vi "old APU + 4 CAMs.vi"() -> ()   [LabVIEW 2013]
uses:
  <vilib>/Platform/TimedLoop/XDataNode/timing_clust.ctl
  <vilib>/Platform/TimedLoop/XDataNode/nitl_modes.ctl
  <vilib>/Platform/TimedLoop/XDataNode/wakeup.ctl
  <userlib>/AES/FPGA/FPGA TypeDefs/aes_FullyCustomTeeth ActionEngine Enum.ctl
  <vilib>/rvi/Emulation/niFpgaSctlEmulationGetInTimedLoop.vi
  <vilib>/rvi/Emulation/niFpgaEmulationReportErrorSimple.vi
  <vilib>/rvi/DataTransferAndStorage/Container/Common/niFpgaContainerGetUniqueNameForEmu.vi
  <vilib>/rvi/DataTransferAndStorage/Container/Common/niFpgaContainerSetEmuInfo.vi
  <vilib>/rvi/eio/common/nirviEmuReportErrorAndStop.vi
  <vilib>/rvi/Emulation/niFpgaGetClockAttributes.vi
  <vilib>/rvi/Emulation/niFpgaCriticalErrorInLSC.vi
  <userlib>/_NI VeriStand FPGA Support/NI VeriStand RIO Library/Custom Device Components/Engine Simulation/Engine Simulation Globals.vi
  <vilib>/rvi/FIFO/Fifo_Resource/nirvififoEmulationReadFpgaImpl.vi
  <vilib>/rvi/eio/common/nirviEmuTemplateMethod_errors.vi
  <vilib>/rvi/Emulation/niFpgaProcessEmulError.vi
  <vilib>/rvi/FIFO/Fifo_Resource/nirvififoEmulationWriteFpgaImpl.vi
  <vilib>/Platform/TimedLoop/XDataNode/XDataNode.xnode
  <vilib>/rvi/LocalResourceManager/LocalResourceManager.xnode
  <vilib>/rvi/DataTransferAndStorage/Container/XNode/niFpgaContainer.xnode
  <vilib>/rvi/FIFO/Fifo_Resource/nirvififoEmulationRead.vi
  <vilib>/eio/EIONode/EIONode.xnode
  <vilib>/rvi/FIFO/Fifo_Resource/nirvififoEmulationWrite.vi
  <vilib>/Platform/TimedLoop/XDataNode/XDNodeRunTimeDep.lvlib
  <userlib>/AES/FPGA/AES FPGA.lvlib
panel:
  in  "FullyCustomTeeth.Cams.Cam1.First Rising?":bool
  in  "FullyCustomTeeth.Cams.Num Angles":u8=2
  in  "FullyCustomTeeth.Cams.Cam1.Offset":u64
  in  "FullyCustomTeeth.Cams.Cam2.Offset":u64
  in  "FullyCustomTeeth.Cams.Cam3.Offset":u64
  in  "FullyCustomTeeth.Cams.Cam4.Offset":u64
  in  "FullyCustomTeeth.Cams.Num Profiles":u8=1
  in  "FullyCustomTeeth.Cams.Cam2.First Rising?":bool
  in  "FullyCustomTeeth.Cams.Cam3.First Rising?":bool
  in  "FullyCustomTeeth.Cams.Cam4.First Rising?":bool
  in  "FullyCustomTeeth.Cams.Cam1.CycleAngle":bool=TRUE
  in  "FullyCustomTeeth.Cams.Cam2.CycleAngle":bool=TRUE
  in  "FullyCustomTeeth.Cams.Cam3.CycleAngle":bool=TRUE
  in  "FullyCustomTeeth.Cams.Cam4.CycleAngle":bool=TRUE
  in  "FullyCustomTeeth.Cams.Data":u64
  in  "FullyCustomTeeth.Cams.Toggle":bool
  in  "APU.Degrees per Tick":u64
  out "APU.Crank Angle":u64
  out "APU.Cycle Angle":u64
  in  "APU.Reset":bool
  in  "APU.Increment Rate":u64
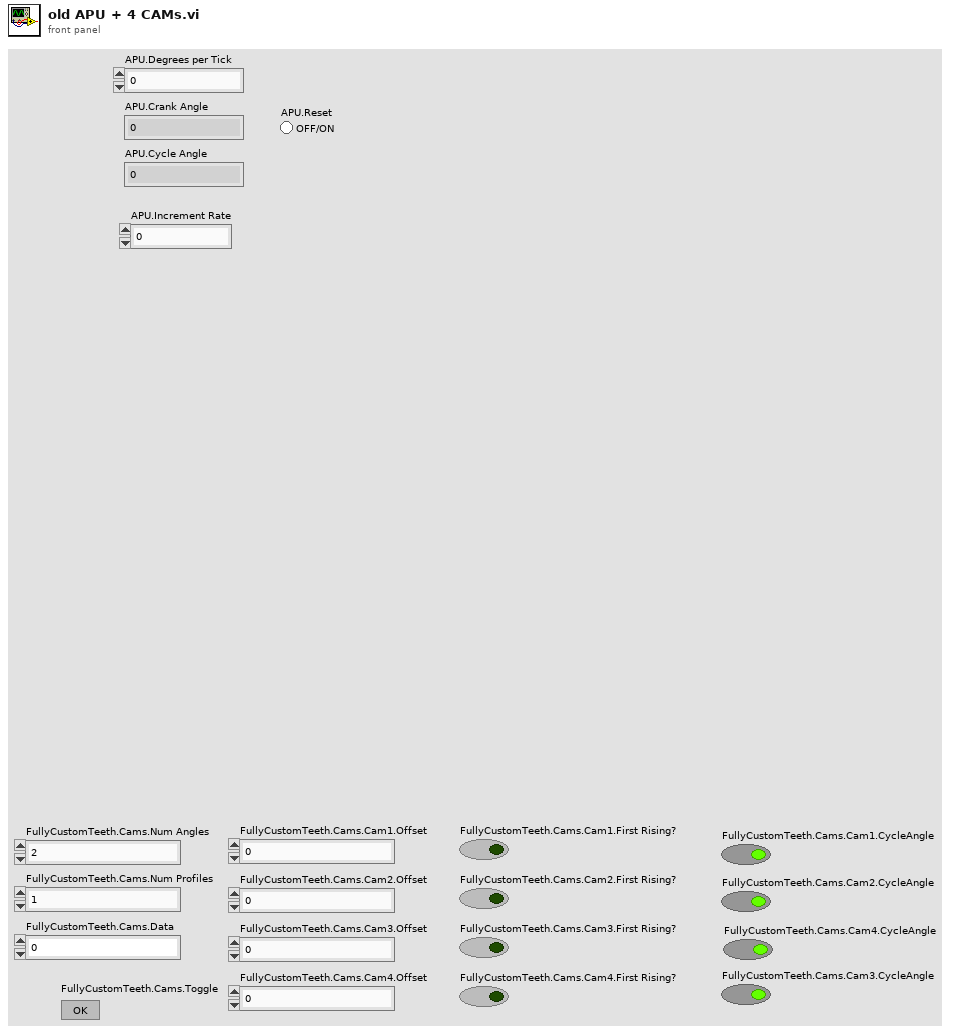
[diagram p1: front panel]
types:
  T1 = typedef "XDNodeRunTimeDep.lvlib/timing_clust.ctl" = cluster{"Expected End [f-1]":u64, "Actual End [f-1]":u64, "Finished Late? [f-1]":bool, "Expected End [i-1]":u64, "Actual End [i-1]":u64, "Finished Late? [i-1]":bool, "Expected Start [i]":u64, "Actual Start [i]":u64, "Expected Start [f]":u64, "Actual Start [f]":u64, "Source Name":string, "Structure Name":string, "Period":i64, "Deadline":i64, "Offset":i64, "Start":i64, "Priority":i32, "Timeout":i32, "Mode":T2, "Wakeup Reason":T3, "Error":errorcluster, "Source Type":string, "Secondary Source Type":string, "Global End Time":u64, "Global Start Time":u64, "Frame Duration":u64, "Iteration Duration":u64, "Assigned CPU":i32, "I/O Scan Engine Mode":u32}
  T2 = typedef "XDNodeRunTimeDep.lvlib/nitl_modes.ctl" = enum32{"No Change", "Process missed periods, maintain original phase", "Discard missed periods, maintain original phase", "Process missed periods, ignore original phase", "Discard missed periods, ignore original phase"}
  T3 = typedef "XDNodeRunTimeDep.lvlib/wakeup.ctl" = enum32{"Normal", "Aborted", "Asynchronous wakeup", "Timing source error", "Timed loop error", "Timeout"}
  T4 = typedef "AES.lvlib/AES FPGA.lvlib/aes_FullyCustomTeeth ActionEngine Enum.ctl" = enum16{"Write Angle", "Update Output"}
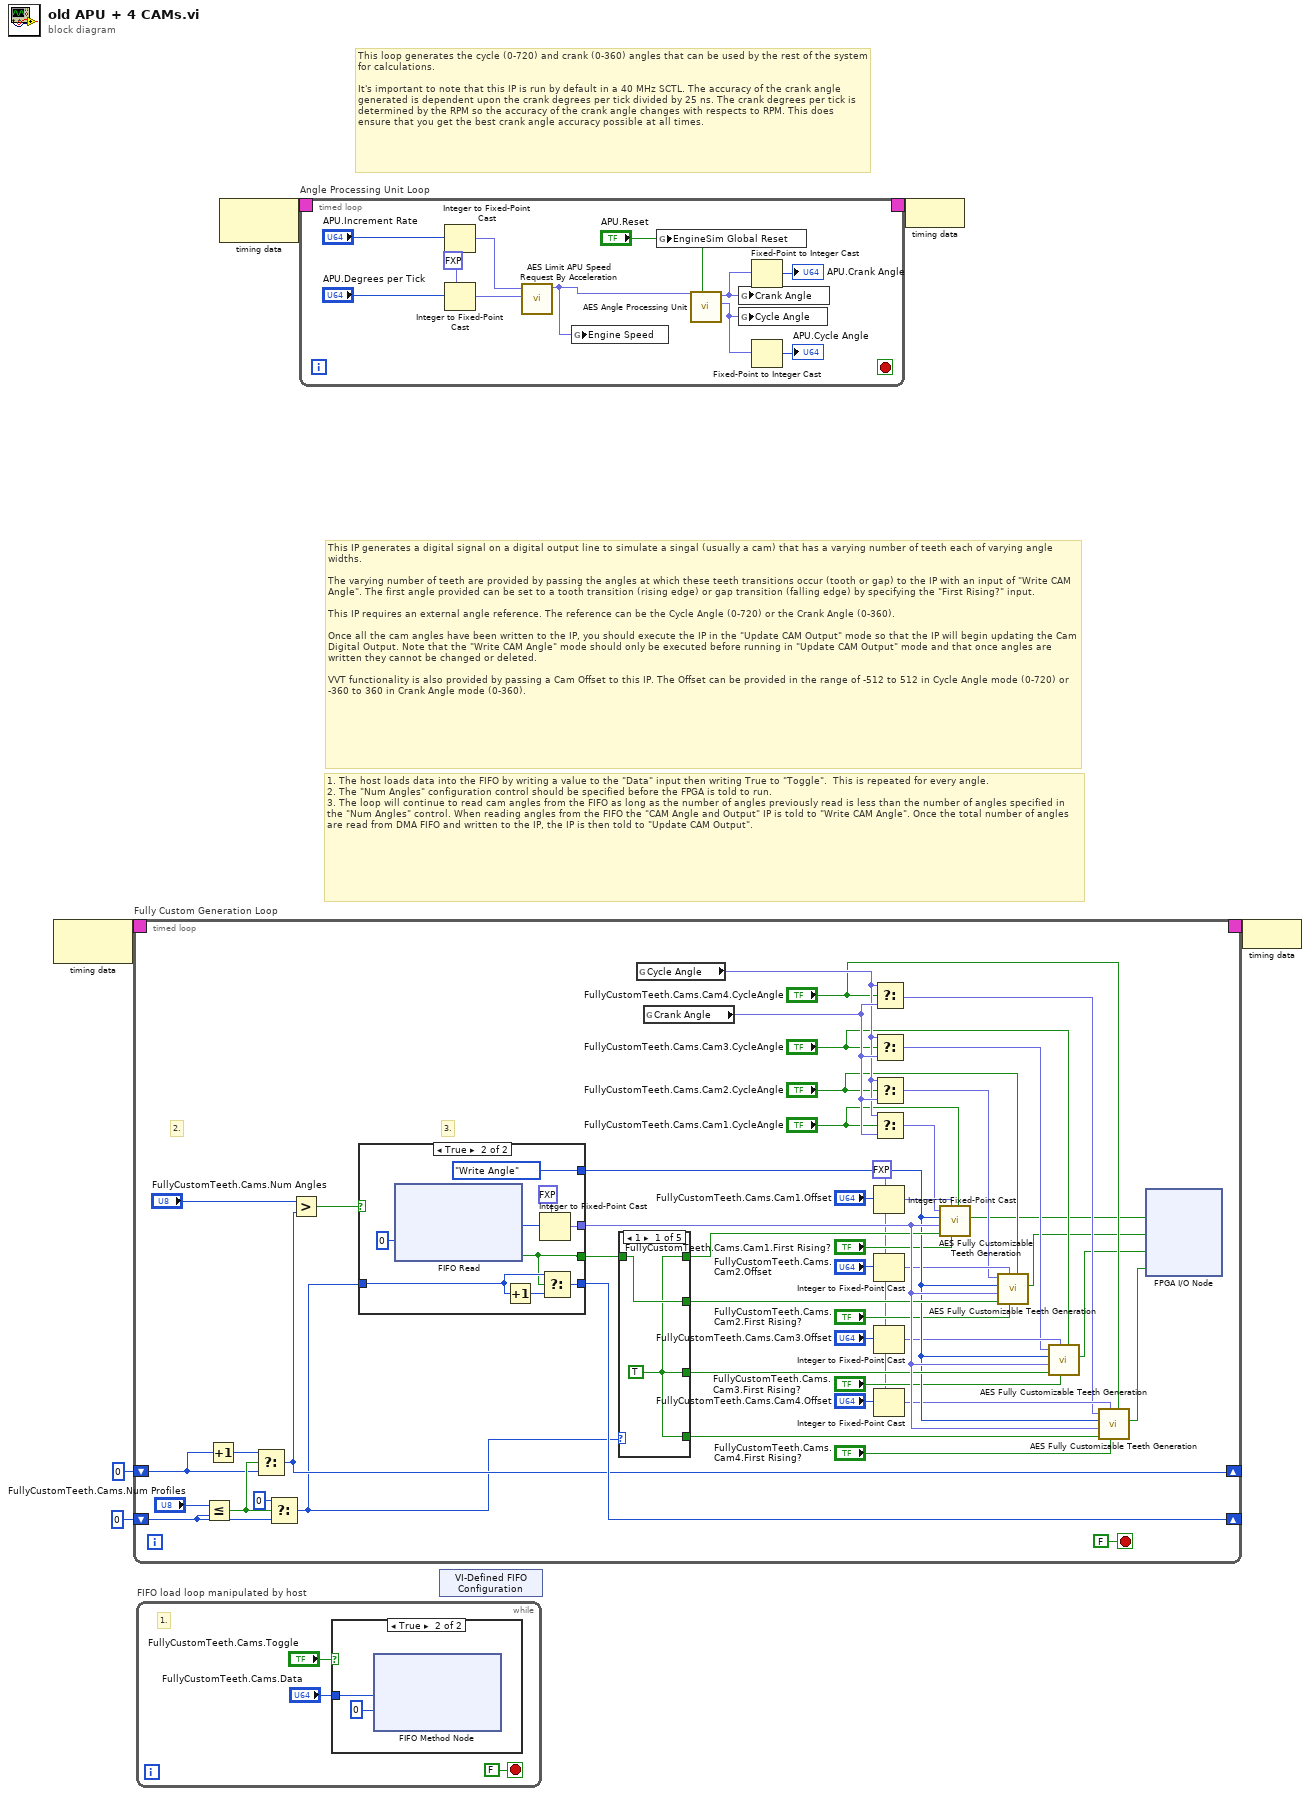
[diagram p0: block diagram]
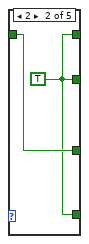
[diagram p3: hidden frame]
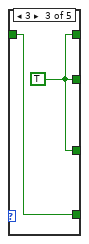
[diagram p4: hidden frame]
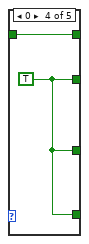
[diagram p5: hidden frame]
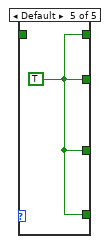
[diagram p6: hidden frame]
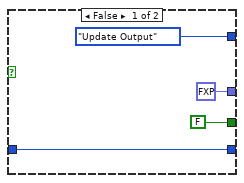
[diagram p7: hidden frame]
diagram:
  # "1. The host loads data into the FIFO by writing a value to the \"Data\" input then writing True to \"Toggle\".  This is repeated for every angle.\n2. The \"Num Angles\" configuration control should be specified before the FPGA is told to run.\n3. The loop will continue to read cam angles from the FIFO as long as the number of angles previously read is less than the number of angles specified in the \"Num Angles\" control. When reading angles from the FIFO the \"CAM Angle and Output\" IP is told to \"Write CAM Angle\". Once the total number of angles are read from DMA FIFO and written to the IP, the IP is then told to \"Update CAM Output\"."
  # "This IP generates a digital signal on a digital output line to simulate a singal (usually a cam) that has a varying number of teeth each of varying angle widths. \n\nThe varying number of teeth are provided by passing the angles at which these teeth transitions occur (tooth or gap) to the IP with an input of \"Write CAM Angle\". The first angle provided can be set to a tooth transition (rising edge) or gap transition (falling edge) by specifying the \"First Rising?\" input. \n\nThis IP requires an external angle reference. The reference can be the Cycle Angle (0-720) or the Crank Angle (0-360). \n\nOnce all the cam angles have been written to the IP, you should execute the IP in the \"Update CAM Output\" mode so that the IP will begin updating the Cam Digital Output. Note that the \"Write CAM Angle\" mode should only be executed before running in \"Update CAM Output\" mode and that once angles are written they cannot be changed or deleted.\n\nVVT functionality is also provided by passing a Cam Offset to this IP. The Offset can be provided in the range of -512 to 512 in Cycle Angle mode (0-720) or -360 to 360 in Crank Angle mode (0-360)."
  # "This loop generates the cycle (0-720) and crank (0-360) angles that can be used by the rest of the system for calculations. \n\nIt's important to note that this IP is run by default in a 40 MHz SCTL. The accuracy of the crank angle generated is dependent upon the crank degrees per tick divided by 25 ns. The crank degrees per tick is determined by the RPM so the accuracy of the crank angle changes with respects to RPM. This does ensure that you get the best crank angle accuracy possible at all times."
  n1 = node-c288() -> (w4:T1)  [unwired: 1 out]
  n2 = timed-loop "Fully Custom Generation Loop" {
    timing: w4 -> [_]
    timing-out: [_] -> w3
    shift-right: [w50] -> _
    shift-left: u8 0 -> [w43]
    shift-right: [w42] -> _
    shift-left: u8 0 ("CAM.Num Angles") -> [w44]
    stop <- FALSE stop-if-true
    w21 = fxp<+/-,61,10> 0.0 ("FullyCustomTeeth.Cams.Cam1.Offset")
    # "3."
    # "2."
    n3 = Less Or Equal?(x="FullyCustomTeeth.Cams.Num Profiles", y=w43) -> (x <= y?=w47:bool)
    n4 = Increment(x=w44) -> (x+1=w46:u8)
    n5 = Select(t=w46, s=w47, f=w44) -> (s? t:f=w42:u8)
    n6 = Select(t=u8 0, s=w47, f=w43) -> (s? t:f=w40:u8)
    n7 = Greater?(x="FullyCustomTeeth.Cams.Num Angles", y=w42) -> (0:w51:bool)
    n8 = case shown="True" w51 {
      tunnel: w40 -> [w65 w72]
      tunnel: [w65 w71] -> w50
      tunnel: [FALSE ("Timed Out?") w70] -> w39
      tunnel: [aes_FullyCustomTeeth_ActionEngine_Enum."Update Output" ("FullyCustomTeeth.Action") aes_FullyCustomTeeth_ActionEngine_Enum."Write Angle" ("FullyCustomTeeth.Action")] -> w34
      tunnel: [fxp<+,61,10> 0.0 ("Element") w67] -> w41
      frame False {
      }
      frame True {
        n9 = xnode ("FIFO Read")("Timeout"=0) -> ("Element"=w69:u64, "Timed Out?"=w70:bool)  [unwired: 1 in, 1 out]
        n10 = Increment(x=w72) -> (x+1=w73:u8)
        n11 = Integer to Fixed-Point Cast(fixed-point type=fxp<+,61,10> 0.0 ("Element"), integer=w69) -> (fixed-point=w67:fxp<+,61,10>)
        n12 = Select(t=w72, s=w70, f=w73) -> (s? t:f=w71:u8)
      }
    }
    n13 = case shown="1" w40 {
      tunnel: w39 -> [w54 w56 w57 w60 _]
      tunnel: [w53 w55 w58 w60 w61] -> w38
      tunnel: [w53 w56 w58 w59 w61] -> w36
      tunnel: [w54 w55 w58 w59 w61] -> w37
      tunnel: [w53 w55 w57 w59 w61] -> w35
      frame 1 {
        w53 = TRUE ("Timed Out?")
      }
      frame 2 {
        w55 = TRUE ("Timed Out?")
      }
      frame 3 {
        w58 = TRUE ("Timed Out?")
      }
      frame 0 {
        w59 = TRUE ("Timed Out?")
      }
      frame Default {
        w61 = TRUE ("Timed Out?")
      }
    }
    n14 = global read "Engine Simulation Globals.vi" "Cycle Angle"() -> (w19:fxp<+,61,10>)
    n15 = global read "Engine Simulation Globals.vi" "Crank Angle"() -> (w20:fxp<+,60,9>)
    n16 = Integer to Fixed-Point Cast(fixed-point type=w21, integer="FullyCustomTeeth.Cams.Cam1.Offset") -> (fixed-point=w28:fxp<+/-,61,10>)
    n17 = Integer to Fixed-Point Cast(fixed-point type=w21, integer="FullyCustomTeeth.Cams.Cam2.Offset") -> (fixed-point=w27:fxp<+/-,61,10>)
    n18 = Integer to Fixed-Point Cast(fixed-point type=w21, integer="FullyCustomTeeth.Cams.Cam3.Offset") -> (fixed-point=w24:fxp<+/-,61,10>)
    n19 = Integer to Fixed-Point Cast(fixed-point type=w21, integer="FullyCustomTeeth.Cams.Cam4.Offset") -> (fixed-point=w22:fxp<+/-,61,10>)
    n20 = Select(t=w19, s="FullyCustomTeeth.Cams.Cam4.CycleAngle", f=w20) -> (s? t:f=w11:fxp<+,61,10>)
    n21 = Select(t=w19, s="FullyCustomTeeth.Cams.Cam3.CycleAngle", f=w20) -> (s? t:f=w14:fxp<+,61,10>)
    n22 = Select(t=w19, s="FullyCustomTeeth.Cams.Cam2.CycleAngle", f=w20) -> (s? t:f=w16:fxp<+,61,10>)
    n23 = Select(t=w19, s="FullyCustomTeeth.Cams.Cam1.CycleAngle", f=w20) -> (s? t:f=w17:fxp<+,61,10>)
    n24 = call <userlib>:"AES Fully Customizable Teeth Generation.vi"("Using Cycle Angle"="FullyCustomTeeth.Cams.Cam1.CycleAngle", "FullyCustomTeeth.FirstElement RisingEdge?"="FullyCustomTeeth.Cams.Cam1.First Rising?", "FullyCustomTeeth.Offset"=w28, "Write Timeout?"=w38, "FullyCustomTeeth.Next Angle"=w41, "FullyCustomTeeth.Action"=w34, "Crank or Cyle Angle"=w17) -> ("FullyCustomTeeth.Digital Output"=w7:bool)  [unwired: 4 in]
    n25 = call <userlib>:"AES Fully Customizable Teeth Generation.vi"("Using Cycle Angle"="FullyCustomTeeth.Cams.Cam2.CycleAngle", "FullyCustomTeeth.FirstElement RisingEdge?"="FullyCustomTeeth.Cams.Cam2.First Rising?", "FullyCustomTeeth.Offset"=w27, "Write Timeout?"=w37, "FullyCustomTeeth.Next Angle"=w41, "FullyCustomTeeth.Action"=w34, "Crank or Cyle Angle"=w16) -> ("FullyCustomTeeth.Digital Output"=w8:bool)  [unwired: 4 in]
    n26 = call <userlib>:"AES Fully Customizable Teeth Generation.vi"("Using Cycle Angle"="FullyCustomTeeth.Cams.Cam3.CycleAngle", "FullyCustomTeeth.FirstElement RisingEdge?"="FullyCustomTeeth.Cams.Cam3.First Rising?", "FullyCustomTeeth.Offset"=w24, "Write Timeout?"=w36, "FullyCustomTeeth.Next Angle"=w41, "FullyCustomTeeth.Action"=w34, "Crank or Cyle Angle"=w14) -> ("FullyCustomTeeth.Digital Output"=w9:bool)  [unwired: 4 in]
    n27 = call <userlib>:"AES Fully Customizable Teeth Generation.vi"("Using Cycle Angle"="FullyCustomTeeth.Cams.Cam4.CycleAngle", "FullyCustomTeeth.FirstElement RisingEdge?"="FullyCustomTeeth.Cams.Cam4.First Rising?", "FullyCustomTeeth.Offset"=w22, "Write Timeout?"=w35, "FullyCustomTeeth.Next Angle"=w41, "FullyCustomTeeth.Action"=w34, "Crank or Cyle Angle"=w11) -> ("FullyCustomTeeth.Digital Output"=w10:bool)  [unwired: 4 in]
    n28 = xnode "FPGA I/O Node"("DO0"=w7, "DO1"=w8, "DO2"=w9, "DO3"=w10) -> ()  [unwired: 4 in, 4 out]
  }
  n29 = while "FIFO load loop manipulated by host" {
    stop <- FALSE stop-if-true
    # "1."
    n30 = case shown="True" "FullyCustomTeeth.Cams.Toggle" {
      tunnel: "FullyCustomTeeth.Cams.Data" -> [_ w81]
      frame False {
      }
      frame True {
        n31 = xnode ("FIFO Method Node")("Element"=w81, "Timeout"=0) -> ()  [unwired: 1 in, 2 out]
      }
    }
  }
  n32 = node-c288() -> (w6:T1)  [unwired: 1 in]
  n33 = timed-loop "Angle Processing Unit Loop" {
    timing: w6 -> [_]
    timing-out: [_] -> w5
    stop <- _ stop-if-true
    w84 = fxp<+/-,47,-4> 0.0 ("Crank.Degrees per Tick")
    n34 = Integer to Fixed-Point Cast(fixed-point type=w84, integer="APU.Increment Rate") -> (fixed-point=w83:fxp<+/-,47,-4>)
    n35 = Integer to Fixed-Point Cast(fixed-point type=w84, integer="APU.Degrees per Tick") -> (fixed-point=w86:fxp<+/-,47,-4>)
    n36 = call <userlib>:"AES Limit APU Speed Request By Acceleration.vi"("APU.Degrees per Tick in"=w86, "APU.Increment Rate"=w83) -> ("APU.Degrees per Tick out"=w82:fxp<+/-,47,-4>)  [unwired: 9 in]
    n37 = global write "Engine Simulation Globals.vi" "Engine Speed"(w82) -> ()
    n38 = global write "Engine Simulation Globals.vi" "EngineSim Global Reset"("APU.Reset") -> ()
    n39 = call <userlib>:"AES Angle Processing Unit.vi"("APU.Reset"="APU.Reset", "APU.Degrees per Tick"=w82) -> ("APU.Cycle Angle"=w88:fxp<+,61,10>, "APU.Crank Angle"=w92:fxp<+,60,9>)  [unwired: 8 in]
    n40 = global write "Engine Simulation Globals.vi" "Crank Angle"(w92) -> ()
    n41 = global write "Engine Simulation Globals.vi" "Cycle Angle"(w88) -> ()
    n42 = Fixed-Point to Integer Cast(1:w92) -> (0:→"APU.Crank Angle":u64)
    n43 = Fixed-Point to Integer Cast(1:w88) -> (0:→"APU.Cycle Angle":u64)
  }
  n44 = xnode "VI-Defined FIFO Configuration"() -> ()  [unwired: 1 out]
  n45 = node-c288(w5) -> ()
  n46 = node-c288(w3) -> ()
